vi "loadInstanceOfEachClassInMemory.vi"() -> (2 "AllClassesInMemory":refnum<class>[](array[class]))   [LabVIEW 2020, in "openg_variant.lvlib" / "ClassLoader.lvclass"]
doc: "GCraftsman JSON Object Serialization Toolkit\nwww.GCraftsman.com\nCopyright (c) 2017, GCraftsman"
uses:
  ClassLoader.lvclass
  ClassLoader.lvclass/ClassLoader.ctl
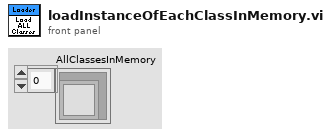
[diagram p1: front panel]
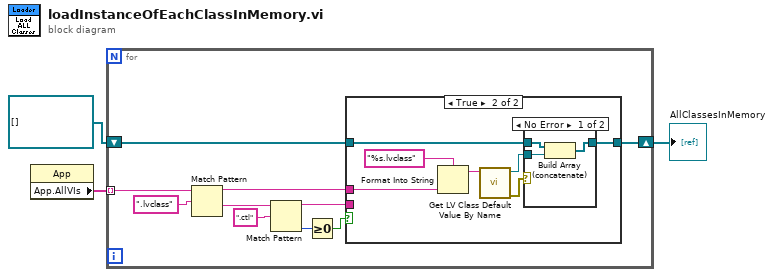
[diagram p0: block diagram]
diagram:
  n1 = property class="App"() -> ("App.AllVIs"=w3:string[])  [unwired: 2 in, 2 out]
  n2 = for {
    tunnel: w3 -> [w13] mode=indexing
    shift-right: [w5] -> w2
    shift-left: refnum<class>[] [] -> [w4]
    n3 = Match Pattern(string=w13, regular expression=".lvclass") -> (before substring=w6:string, after substring=w11:string)  [unwired: 1 in, 2 out]
    n4 = Match Pattern(string=w11, regular expression=".ctl") -> (before substring=w7:string, offset past match=w9:i32)  [unwired: 1 in, 2 out]
    n5 = Greater Or Equal To 0?(x=w9) -> (x >= 0?=w8:bool)
    n6 = case shown="True" w8 {
      tunnel: w6 -> [_ w19]
      tunnel: w7 -> [_ _]
      tunnel: [w14 w21] -> w5
      tunnel: w4 -> [w14 w20]
      frame False {
      }
      frame True {
        n7 = Format Into String(format string="%s.lvclass", w19) -> (resulting string=w16:string)  [unwired: 2 in, 1 out]
        n8 = call <vilib>:"Get LV Class Default Value By Name.vi"("class name"=w16) -> ("error out"=w17:errorcluster, "object"=w15:refnum<class>)  [unwired: 9 in]
        n9 = case shown="No Error" w17 {
          tunnel: w15 -> [w24 _]
          tunnel: [w23 w25] -> w21
          tunnel: w20 -> [w22 w25]
          frame No Error {
            n10 = Build Array (concatenate)(w22, w24) -> (w23:refnum<class>[])
          }
          frame Error {
          }
        }
      }
    }
  }
  "AllClassesInMemory" <- w2
